vi "System Explorer - Copy Templates for System Explorer.vi"(7 "CD Name":string, 8 "error in (no error)":errorcluster, 10 "CD Template":refnum<class "NIVS_CD Template.lvclass">, 11 "System Explorer folder":path) -> (0 "error out":errorcluster)   [LabVIEW 2020, in "NIVS_Consolidated_CDW_MetaDataObj.lvclass"]
doc: "Copy the templates for the System Explorer library into the System Explorer folder and disconnect the templates from the owning library."
uses:
  NIVS_Consolidated_CDW_MetaDataObj.lvclass
  Template Classes/NIVS_CD Template/NIVS_CD Template.lvclass
  CD System Explorer lvlib.ctl
  Common.ctl
  CD Shared lvlib.ctl
  Template Classes/NIVS_CD Template/NIVS_CD Template.lvclass/NIVS_CD Template.ctl
  Template Classes/NIVS_CD Template/Read Support Runtime Configuration.vi
  CD System Explorer lvlib.vi
  Common.vi
  CD Shared lvlib.vi
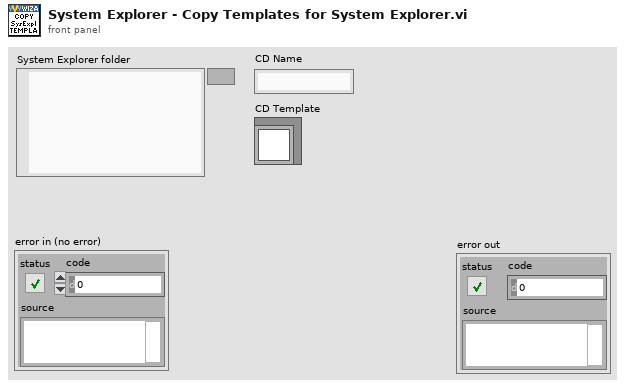
[diagram p1: front panel]
types:
  T1 = typedef "NIVS_Consolidated_CDW_MetaDataObj.lvclass/CD Shared lvlib.ctl" = enum16{"LibraryFileName", "LibraryFolderName", "ConstantsVI.VIPathAndName", "Shared.FolderName", "Shared.Types.FolderName", "Shared.Constants.VIName", "Shared.Constants.VITemplateName", "Shared.Constants.VITemplatePathAndName", "Shared.CompiledSettings.RelativePath", "Shared.Constants.RelativePath", "Shared.CompiledSettings.Name", "Shared.CompiledSettings.Name.NoExtension", "Shared.CompiledSettings.ClusterName"}
  T2 = typedef "NIVS_Consolidated_CDW_MetaDataObj.lvclass/CD System Explorer lvlib.ctl" = enum16{"LibraryFileName", "LibraryFolderName", "System Explorer.FolderName", "System Explorer.Dynamically Called.FolderName", "System Explorer.Dynamically Called.Extra Pages.FolderName", "System Explorer.Dynamically Called.Extra Pages.TemplatePathAndName", "System Explorer.Dynamically Called.Main Page.VIName", "System Explorer.Dynamically Called.Main Page.TemplatePathAndName", "System Explorer.Dynamically Called.Initialization VI.VIName", "System Explorer.Dynamically Called.Initialization VI.TemplatePathAndName", "System Explorer.SubVI.FolderName", "System Explorer.Types.FolderName", "System Explorer.ActionVIOnCompile.VIName", "System Explorer.ActionVIOnRecompile.VIName", "System Explorer.ExportConfigRTM.VIName", "System Explorer.PPL.ExportConfigRTM.VIName", "System Explorer.LoadHelpFile.VIName", "System Explorer.PPL.LoadHelpFile.VIName", "System Explorer.SetRTDriverVIsFilePaths.VIName", "System Explorer.ClearRTDriverVIs.VIName"}
  T3 = typedef "NIVS_Consolidated_CDW_MetaDataObj.lvclass/Common.ctl" = enum16{"ProjectName", "TemplatesFolderName", "PPLTemplatesFolderName", "ProjectTemplatePathAndName", "ProjectPPLTemplatePathAndName", "TimingAndSyncFolderName", "CustomDeviceFolderName", "PathToTemplates", "PathToPPLTemplates", "PathToExplorerPPLTemplates", "PathToEnginePPLTemplates", "PathToConfigurationFile", "ProjectConfigurationName"}
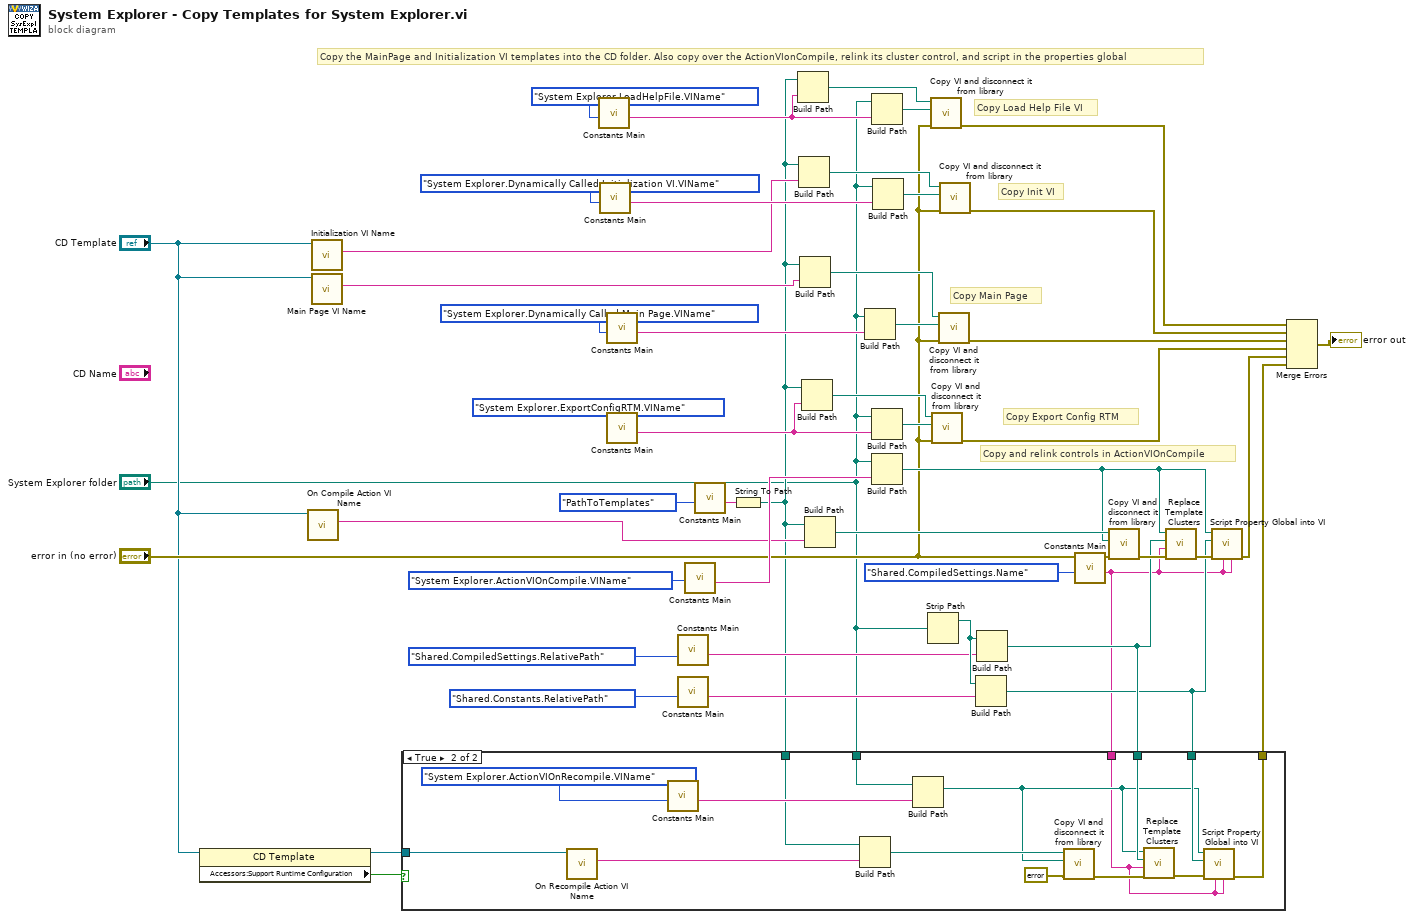
[diagram p0: block diagram]
diagram:
  # "Copy Load Help File VI"
  # "Copy the MainPage and Initialization VI templates into the CD folder. Also copy over the ActionVIonCompile, relink its cluster control, and script in the properties global"
  # "Copy Export Config RTM"
  # "Copy and relink controls in ActionVIOnCompile"
  # "Copy Main Page"
  # "Copy Init VI"
  n1 = property class="CD Template"(reference="CD Template") -> (reference out=w9:refnum<class "NIVS_CD Template.lvclass">, "Accessors:Support Runtime Configuration"=w8:bool)  [unwired: 1 in, 1 out]
  n2 = call-dynamic "On Compile Action VI Name.vi"("CD Template in"="CD Template") -> ("On Compile Action VI Name"=w12:string)  [unwired: 10 in]
  n3 = call-dynamic "Initialization VI Name.vi"("CD Template in"="CD Template") -> ("Initialization VI Name"=w14:string)  [unwired: 10 in]
  n4 = call-dynamic "Main Page VI Name.vi"("CD Template in"="CD Template") -> ("Main Page VI Name"=w13:string)  [unwired: 10 in]
  n5 = call-poly "Constants Main.vi"("Action"=CD_System_Explorer_lvlib."System Explorer.LoadHelpFile.VIName") -> ("Output"=w20:string)  [unwired: 10 in]
  n6 = call-poly "Constants Main.vi"("Action"=CD_System_Explorer_lvlib."System Explorer.Dynamically Called.Initialization VI.VIName") -> ("Output"=w38:string)  [unwired: 10 in]
  n7 = call-poly "Constants Main.vi"("Action"=CD_System_Explorer_lvlib."System Explorer.Dynamically Called.Main Page.VIName") -> ("Output"=w37:string)  [unwired: 10 in]
  n8 = call-poly "Constants Main.vi"("Action"=CD_System_Explorer_lvlib."System Explorer.ExportConfigRTM.VIName") -> ("Output"=w25:string)  [unwired: 10 in]
  n9 = call-poly "Constants Main.vi"("Action"=CD_Shared_lvlib."Shared.CompiledSettings.RelativePath") -> ("Output"=w10:string)  [unwired: 10 in]
  n10 = call-poly "Constants Main.vi"("Action"=CD_Shared_lvlib."Shared.Constants.RelativePath") -> ("Output"=w30:string)  [unwired: 10 in]
  n11 = call-poly "Constants Main.vi"("Action"=CD_System_Explorer_lvlib."System Explorer.ActionVIOnCompile.VIName") -> ("Output"=w32:string)  [unwired: 10 in]
  n12 = call-poly "Constants Main.vi"("Action"=Common."PathToTemplates") -> ("Output"=w43:string)  [unwired: 10 in]
  n13 = String To Path(string=w43) -> (path=w3:path)
  n14 = Build Path(base path=w3, name or relative path=w20) -> (appended path=w19:path)
  n15 = Build Path(base path=w3, name or relative path=w14) -> (appended path=w39:path)
  n16 = Build Path(base path=w3, name or relative path=w13) -> (appended path=w40:path)
  n17 = Build Path(base path=w3, name or relative path=w25) -> (appended path=w28:path)
  n18 = Build Path(base path=w3, name or relative path=w12) -> (appended path=w42:path)
  n19 = Build Path(base path="System Explorer folder", name or relative path=w37) -> (appended path=w21:path)
  n20 = Build Path(base path="System Explorer folder", name or relative path=w20) -> (appended path=w18:path)
  n21 = Build Path(base path="System Explorer folder", name or relative path=w25) -> (appended path=w27:path)
  n22 = Build Path(base path="System Explorer folder", name or relative path=w32) -> (appended path=w35:path)
  n23 = Build Path(base path="System Explorer folder", name or relative path=w38) -> (appended path=w46:path)
  n24 = Strip Path(path="System Explorer folder") -> (stripped path=w34:path)  [unwired: 1 out]
  n25 = call "Copy VI and disconnect it from library.vi"("error in (no error)"="error in (no error)", "VI Target Path"=w18, "VI Source Path"=w19) -> ("error out"=w16:errorcluster)  [unwired: 8 in]
  n26 = call "Copy VI and disconnect it from library.vi"("error in (no error)"="error in (no error)", "VI Target Path"=w27, "VI Source Path"=w28) -> ("error out"=w23:errorcluster)  [unwired: 8 in]
  n27 = call "Copy VI and disconnect it from library.vi"("error in (no error)"="error in (no error)", "VI Target Path"=w21, "VI Source Path"=w40) -> ("error out"=w22:errorcluster)  [unwired: 8 in]
  n28 = call "Copy VI and disconnect it from library.vi"("error in (no error)"="error in (no error)", "VI Target Path"=w46, "VI Source Path"=w39) -> ("error out"=w45:errorcluster)  [unwired: 8 in]
  n29 = Build Path(base path=w34, name or relative path=w30) -> (appended path=w4:path)
  n30 = Build Path(base path=w34, name or relative path=w10) -> (appended path=w5:path)
  n31 = call-poly "Constants Main.vi"("Action"=CD_Shared_lvlib."Shared.CompiledSettings.Name") -> ("Output"=w1:string)  [unwired: 10 in]
  n32 = case shown="True" w8 {
    tunnel: w9 -> [_ w64]
    tunnel: w4 -> [_ w60]
    tunnel: w5 -> [_ w59]
    tunnel: [_ w54] -> w7
    tunnel: w3 -> [_ w51]
    tunnel: "System Explorer folder" -> [_ w52]
    tunnel: w1 -> [_ w50]
    frame False {
    }
    frame True {
      n33 = call-dynamic "On Recompile Action VI Name.vi"("CD Template in"=w64) -> ("On Recompile Action VI Name"=w63:string)  [unwired: 10 in]
      n34 = call-poly "Constants Main.vi"("Action"=CD_System_Explorer_lvlib."System Explorer.ActionVIOnRecompile.VIName") -> ("Output"=w61:string)  [unwired: 10 in]
      n35 = Build Path(base path=w51, name or relative path=w63) -> (appended path=w58:path)
      n36 = Build Path(base path=w52, name or relative path=w61) -> (appended path=w57:path)
      n37 = call "Copy VI and disconnect it from library.vi"("error in (no error)"=errorcluster {"status"=FALSE, "code"=0, "source"=""}, "VI Target Path"=w57, "VI Source Path"=w58) -> ("error out"=w56:errorcluster)  [unwired: 8 in]
      n38 = call "Replace Template Clusters.vi"("error in (no error)"=w56, "Control Name"=w50, "Path to Cluster to Replace"=w59, "Path to VI"=w57) -> ("error out"=w55:errorcluster)  [unwired: 7 in]
      n39 = call "Script Property Global into VI.vi"("GlobalControlName"=w50, "StringConstantToReplace"=w50, "error in (no error)"=w55, "Path to Global"=w60, "Path to VI"=w57) -> ("error out"=w54:errorcluster)  [unwired: 6 in]
    }
  }
  n40 = call "Copy VI and disconnect it from library.vi"("error in (no error)"="error in (no error)", "VI Target Path"=w35, "VI Source Path"=w42) -> ("error out"=w41:errorcluster)  [unwired: 8 in]
  n41 = call "Replace Template Clusters.vi"("error in (no error)"=w41, "Control Name"=w1, "Path to Cluster to Replace"=w5, "Path to VI"=w35) -> ("error out"=w36:errorcluster)  [unwired: 7 in]
  n42 = call "Script Property Global into VI.vi"("GlobalControlName"=w1, "StringConstantToReplace"=w1, "error in (no error)"=w36, "Path to Global"=w4, "Path to VI"=w35) -> ("error out"=w24:errorcluster)  [unwired: 6 in]
  n43 = Merge Errors(w16, w45, w22, w23, w24, w7) -> (→"error out":errorcluster)
